vi "DataTree_Add_Crv_Names.vi"(0 "référence":refnum<vi>, 5 "Parent Name":string, 7 "Scan list":string[](array[string]), 9 "Time":string, 11 "Entrée d'erreur":errorcluster, 12 "NbPoint":string, 13 "FileIndex":i32) -> (4 "Tag Courbes":string[](array[string]), 15 "Sortie d'erreur":errorcluster)   [LabVIEW 2019]
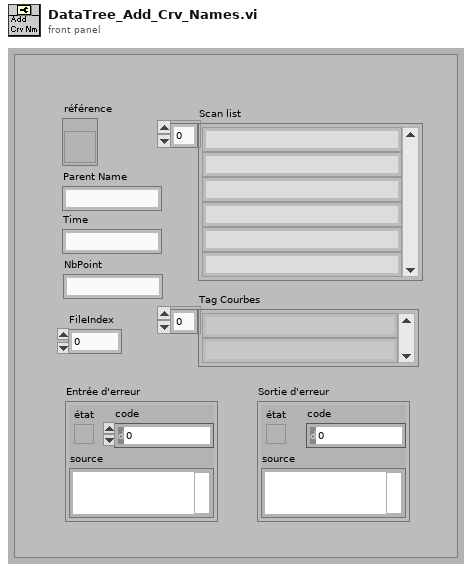
[diagram p1: front panel]
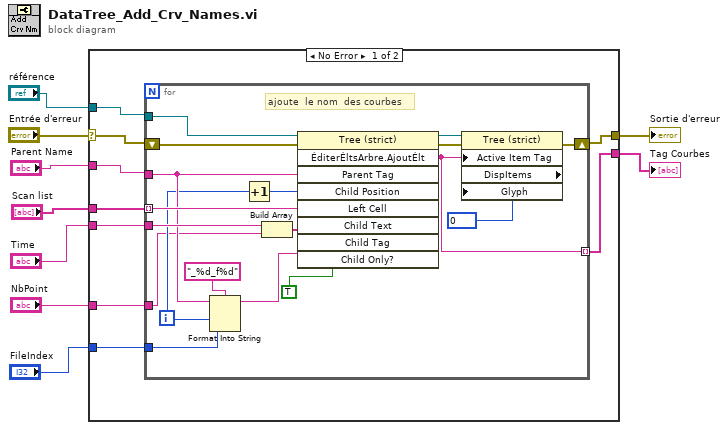
[diagram p0: block diagram]
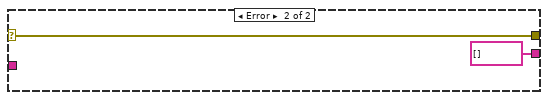
[diagram p2: hidden frame]
diagram:
  n1 = case shown="No Error" "Entrée d'erreur" {
    selector: "Entrée d'erreur" -> [w17 w38]
    tunnel: [w18 w38] -> w9
    tunnel: "Parent Name" -> [w16 _]
    tunnel: "Scan list" -> [w15 _]
    tunnel: "Time" -> [w14 _]
    tunnel: "référence" -> [w13 _]
    tunnel: [w12 string[] []] -> w3
    tunnel: "NbPoint" -> [w11 _]
    tunnel: "FileIndex" -> [w10 _]
    frame No Error {
      n2 = for {
        tunnel: w16 -> [w30]
        tunnel: w15 -> [w35] mode=indexing
        tunnel: w14 -> [w34]
        shift-right: [w23] -> w18
        shift-left: w17 -> [w27]
        tunnel: w13 -> [w26]
        tunnel: [w22] -> w12 mode=indexing
        tunnel: w11 -> [w20]
        tunnel: w10 -> [w19]
        i -> [w28]
        # "ajoute  le nom  des courbes"
        n3 = Format Into String(format string="_%d_f%d" ("chaîne de format"), initial string=w30, w28, w19) -> (resulting string=w29:string)  [unwired: 1 in, 1 out]
        n4 = Increment(x=w28) -> (x+1=w36:i32)
        n5 = Build Array(w34, w20) -> (w33:string[])
        n6 = invoke on="Nœud de méthode" class="Tree (strict)" method="ÉditerÉltsArbre.AjoutÉlt"(reference=w26, error in=w27, "Parent Tag"=w30, "Child Position"=w36, "Left Cell"=w35, "Child Text"=w33, "Child Tag"=w29, "Child Only?"=TRUE ("Enfant uniquement ?")) -> (reference out=w25:refnum<vi>, error out=w24:errorcluster, "Edit Tree Items:Add Item"=w22:string)  [unwired: 1 in, 6 out]
        n7 = property on="Nœud de propriété" class="Tree (strict)" props=["Active Item Tag", "DispItems", "Glyph"](reference=w25, error in=w24, "Active Item Tag"=w22, "Glyph"=0) -> (error out=w23:errorcluster)  [unwired: 2 out]
      }
    }
    frame Error {
    }
  }
  "Sortie d'erreur" <- w9
  "Tag Courbes" <- w3
